vi "Gyro PID Fwd C2 Assisted - Left Edge.vi"(5 "Target reflection":sgl=32.0, 6 "Target angle":sgl, 7 "Threshold to Color":i32=600, 8 "Threshold to slow":i32=400, 9 "Min. speed":i32=20, 10 "Max. speed":i32=40, 11 "EV3 in":T1) -> (3 "EV3 out":T1)   [LabVIEW 2016]
uses:
  <vilib>/NXT/Subs/LVHSConnector.ctl
  <vilib>/NXT/LegoClasses/BrickReference/BrickReference.lvclass
  <vilib>/NXT/Block Support/NXT_OutputPort.ctl
  <vilib>/NXT/Block Support/NXT_InputPort.ctl
  <vilib>/NXT/NXTIO Xnodes/NXTIONodeSubVIs/LEGOResetMotors.vi
  <vilib>/NXT/Dual Mode Library/Motors/Rotation.vi
  <vilib>/NXT/Dual Mode Library/Sensors/EV3_Color_Reflect.vi
  <vilib>/NXT/NXTIO Xnodes/NXTIONodeSubVIs/NXTMotorSteeringOn.vi
  <vilib>/NXT/NXTIO Xnodes/NXTIONodeSubVIs/NXTStopMotors.vi
  <vilib>/NXT/Dual Mode Library/Waits/Wait_Num.vi
  <vilib>/NXT/NXTIO Xnodes/NXTIOXNode/NXTIO.xnode
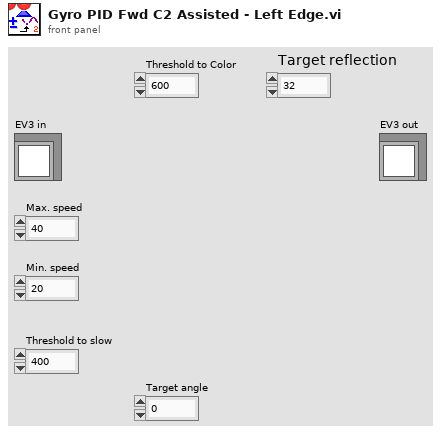
[diagram p1: front panel]
types:
  T1 = typedef "LVHSConnector.ctl" = refnum<class "BrickReference.lvclass">
  T2 = typedef "NXT_OutputPort.ctl" = u8
  T3 = typedef "NXT_InputPort.ctl" = u32
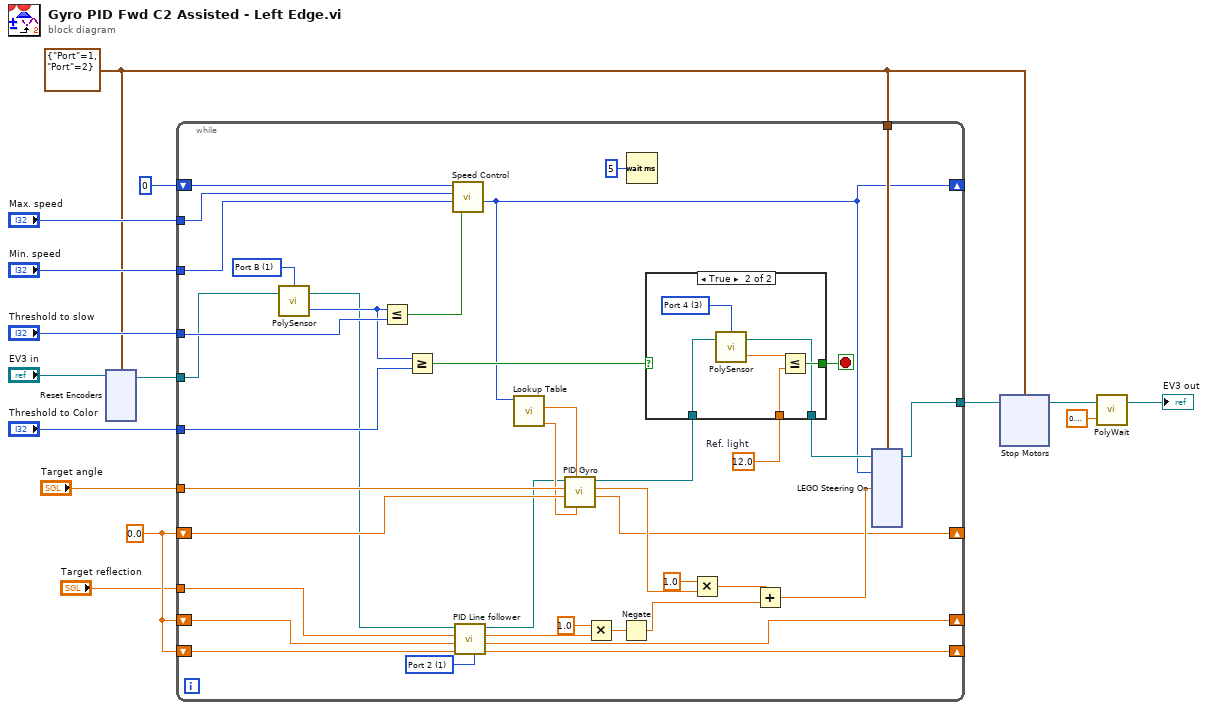
[diagram p0: block diagram]
diagram:
  w6 = cluster{"Port":T2, "Port":T2} {"Port"=1, "Port"=2} ("Motor")
  w2 = sgl 0.0
  n1 = xnode "Reset Encoders"("Motors"=w6, "NXT/EV3"="EV3 in") -> ("NXT/EV3"=w12:T1)
  n2 = while {
    tunnel: w12 -> [w45]
    shift-right: [w20] -> _
    shift-left: w2 -> [w42]
    tunnel: "Target angle" -> [w54]
    tunnel: [w51] -> w8
    tunnel: w6 -> [w53]
    shift-right: [w33] -> _
    shift-left: 0 -> [w49]
    tunnel: "Min. speed" -> [w46]
    tunnel: "Max. speed" -> [w48]
    tunnel: "Threshold to slow" -> [w47]
    tunnel: "Threshold to Color" -> [w41]
    shift-right: [w26] -> _
    shift-left: w2 -> [w30]
    shift-right: [w27] -> _
    shift-left: w2 -> [w28]
    tunnel: "Target reflection" -> [w24]
    stop <- w40 stop-if-true
    w17 = T3 1 items=["Port 1", "Port 2", "Port 3", "Port 4"] ("Port (Port 1)")
    w36 = sgl 12.0  # Ref. light
    w52 = T2 1 items=["Port A", "Port B", "Port C", "Port D"] ("Port (Port A)")
    n3 = call-poly <vilib>:"PolySensor.vi"("NXT/EV3"=w45, "Port (Port A)"=w52) -> ("Angle of Rotation"=w43:i32, "NXT/EV3"=w23:T1)  [unwired: 1 in]
    n4 = Less Or Equal?(x=w43, y=w47) -> (x <= y?=w44:bool)
    n5 = Greater Or Equal?(x=w43, y=w41) -> (x >= y?=w39:bool)
    n6 = call "Speed Control.vi"("Speed Up or Down?"=w44, "Min. speed"=w46, "Max. speed"=w48, "Ini. speed"=w49) -> ("Speed out"=w33:i32)  [unwired: 7 in]
    n7 = call "PID Line follower.vi"("Port (Port 1)"=w17, "Old Error"=w30, "Previous integral"=w28, "Target reflection"=w24, "EV3 in"=w23) -> ("New Error"=w26:sgl, "New integral"=w27:sgl, "Total error"=w25:sgl, "EV3 out"=w29:T1)  [unwired: 3 in]
    n8 = call "Lookup Table.vi"("Speed"=w33) -> ("I"=w31:dbl, "P"=w32:dbl)  [unwired: 9 in]
    n9 = call "PID Gyro.vi"("K_i"=w31, "K_p"=w32, "Previous integral"=w42, "Target angle"=w54, "EV3 in"=w29) -> ("New integral"=w20:sgl, "Total error"=w35:sgl, "EV3 out"=w38:T1)  [unwired: 4 in]
    n10 = Multiply(x=sgl 1.0, y=w25) -> (x*y=w22:sgl)
    n11 = Negate(x=w22) -> (-x=w16:sgl)
    n12 = Wait (ms)(milliseconds to wait=u32 5) -> ()  [unwired: 1 out]
    n13 = case shown="True" w39 {
      tunnel: [_ w59] -> w40
      tunnel: w38 -> [w55 w58]
      tunnel: [w55 w57] -> w37
      tunnel: w36 -> [_ w56]
      frame False {
      }
      frame True {
        w61 = T3 3 items=["Port 1", "Port 2", "Port 3", "Port 4"] ("Port (Port 1)")
        n14 = call-poly <vilib>:"PolySensor.vi"("NXT/EV3"=w58, "Port (Port 1)"=w61) -> ("Scaled Value"=w60:sgl, "NXT/EV3"=w57:T1)  [unwired: 1 in]
        n15 = Less Or Equal?(x=w60, y=w56) -> (x <= y?=w59:bool)
      }
    }
    n16 = Multiply(x=sgl 1.0, y=w35) -> (x*y=w19:sgl)
    n17 = Add(x=w19, y=w16) -> (x+y=w34:sgl)
    n18 = xnode "LEGO Steering On"("Steering 1"=w34, "Power 1"=w33, "Motors"=w53, "NXT/EV3"=w37) -> ("NXT/EV3"=w51:T1)
  }
  n19 = xnode "Stop Motors"("Motors"=w6, "NXT/EV3"=w8) -> ("NXT/EV3"=w7:T1)
  n20 = call-poly <vilib>:"PolyWait.vi"("Time (1 sec)"=sgl 0.2, "NXT/EV3"=w7) -> ("NXT/EV3"=→"EV3 out":T1)  [unwired: 2 in]
